vi "Poly Set Map List Data Types.vi"(11 "Poly Set Map":T1) -> (3 "Data Types":string[][](array[string]))   [LabVIEW 2020]
uses:
  e8a105fa-0b4f-4f6c-a7d8-1dcfe4b15b18.vi
  _td_cluster_InstanceInfo.ctl
  _td_map_PolyInstanceInfo.ctl
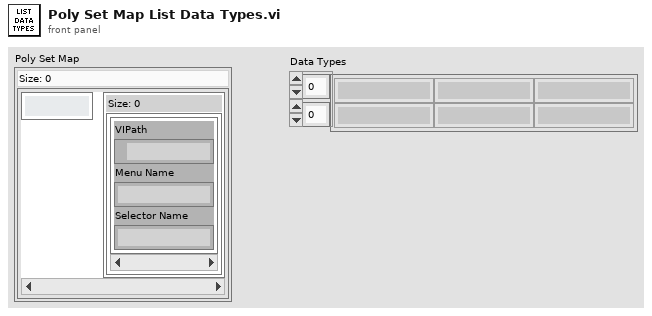
[diagram p1: front panel]
types:
  T1 = typedef "_td_map_PolyInstanceInfo.ctl" = map{string, set{T2}}
  T2 = typedef "_td_cluster_InstanceInfo.ctl" = cluster{"VIPath":path, "Menu Name":string, "Selector Name":string}
  T3 = map{string, set{cluster{"VIPath":path, "Menu Name":string, "Selector Name":string}}}
  T4 = set{cluster{"VIPath":path, "Menu Name":string, "Selector Name":string}}
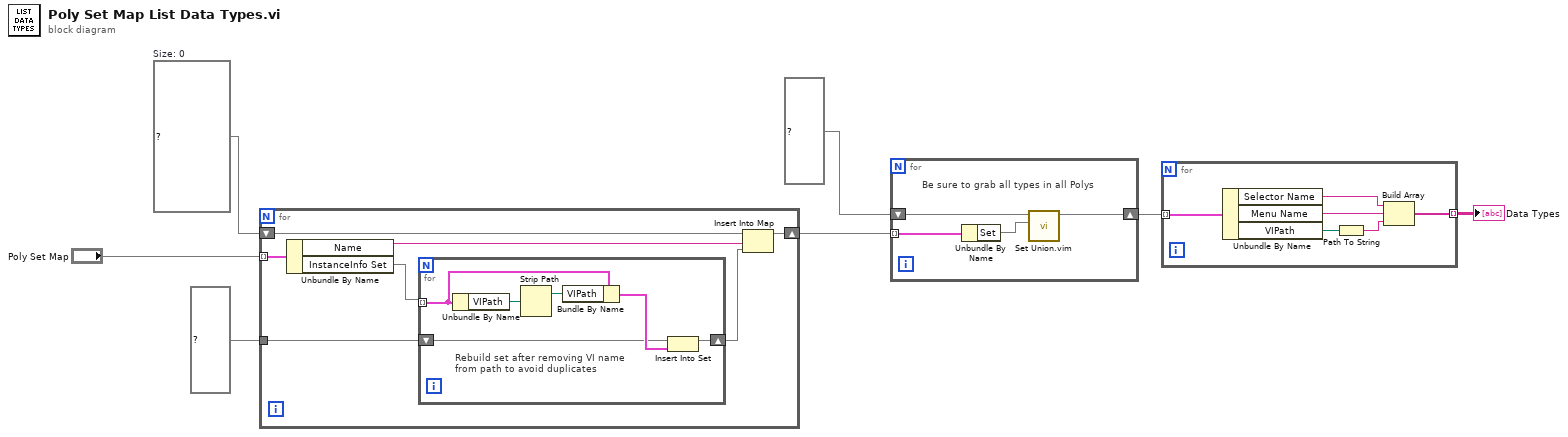
[diagram p0: block diagram]
diagram:
  w2 = T3 {}  # Size: 0
  n1 = for {
    tunnel: "Poly Set Map" -> [w14] mode=indexing
    tunnel: T4 {} ("Set") -> [w11]
    shift-right: [w9] -> w3
    shift-left: w2 -> [w8]
    n2 = Unbundle By Name(w14) -> ("Name"=w12:string, "InstanceInfo Set"=w13:set{T2})
    n3 = for {
      tunnel: w13 -> [w19] mode=indexing
      shift-right: [w16] -> w10
      shift-left: w11 -> [w15]
      # "Rebuild set after removing VI name \nfrom path to avoid duplicates"
      n4 = Unbundle By Name(w19) -> ("VIPath"=w20:path)
      n5 = Strip Path(path=w20) -> (stripped path=w18:path)  [unwired: 1 out]
      n6 = Bundle By Name(cluster=w19, "VIPath"=w18) -> (w17:T2)
      n7 = Insert Into Set(10:w17, 11:w15) -> (3:w16:T4)  [unwired: 1 out]
    }
    n8 = Insert Into Map(map in=w8, key=w12, value=w10) -> (map out=w9:T3)  [unwired: 2 out]
  }
  n9 = for {
    tunnel: w3 -> [w22] mode=indexing
    shift-right: [w24] -> w7
    shift-left: T4 {} ("Set") -> [w23]
    # "Be sure to grab all types in all Polys"
    n10 = Unbundle By Name(w22) -> ("Set"=w21:T4)
    n11 = call "Set Union.vim"("set 2"=w21, "set 1"=w23) -> ("union"=w24:T4)  [unwired: 9 in]
  }
  n12 = for {
    tunnel: w7 -> [w30] mode=indexing
    tunnel: [w25] -> w5 mode=indexing
    n13 = Unbundle By Name(w30) -> ("Selector Name"=w29:string, "Menu Name"=w28:string, "VIPath"=w27:path)
    n14 = Path To String(path=w27) -> (string=w26:string)
    n15 = Build Array(w29, w28, w26) -> (w25:string[])
  }
  "Data Types" <- w5
